vi "Get Data Logging Session Names.vi"(8 "error in (no error)":errorcluster, 11 "Data Logging Manager Ref in":T1) -> (0 "error out":errorcluster, 2 "Session Names":string[](array[string]), 3 "Data Logging Manager Ref out":T1)   [LabVIEW 2020, in "NI_VS Data Logging API.lvlib"]
doc: "Returns the names of the currently active data logging sessions in the VeriStand Gateway."
uses:
  <vilib>/NI VeriStand/Execution/DataLogging/NI_VS Data Logging API.lvlib
  <vilib>/NI VeriStand/Execution/DataLogging/IDataLogging Ref.ctl
  NationalInstruments.VeriStand.ClientAPI
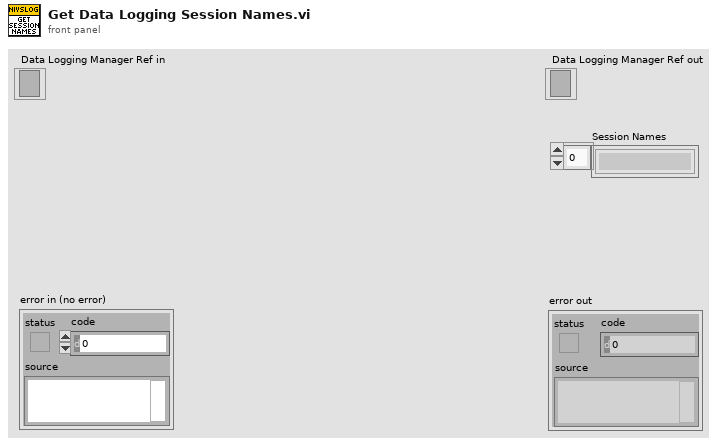
[diagram p1: front panel]
types:
  T1 = typedef "NI_VS Data Logging API.lvlib/IDataLogging Ref.ctl" = refnum<k24>
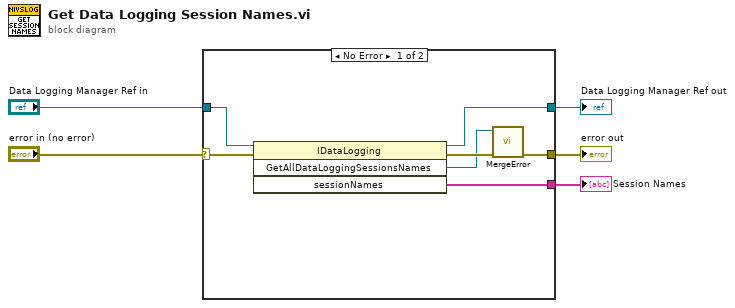
[diagram p0: block diagram]
diagram:
  n1 = case shown="No Error" "error in (no error)" {
    selector: "error in (no error)" -> [w11 w14]
    tunnel: [w8 w14] -> w4
    tunnel: [w7 w13] -> w3
    tunnel: "Data Logging Manager Ref in" -> [w12 w13]
    tunnel: [w6 _] -> w1
    frame No Error {
      n2 = invoke class="IDataLogging" method="GetAllDataLoggingSessionsNames"(reference=w12, error in=w11) -> (reference out=w7:T1, error out=w10:errorcluster, "GetAllDataLoggingSessionsNames"=w9:refnum<k24>, "sessionNames"=w6:string[])  [unwired: 2 in]
      n3 = call <vilib>:"MergeError.vi"("error in (no error)"=w10, "Error"=w9) -> ("error out"=w8:errorcluster)  [unwired: 9 out]
    }
    frame Error {
    }
  }
  "Data Logging Manager Ref out" <- w3
  "error out" <- w4
  "Session Names" <- w1
